vi "Network Parameters DAO.vi"(5 "Section":string="DataTransmission", 7 "refnum":T2, 8 "error in (no error)":errorcluster, 10 "Network Parameters In":T1={"Port Number"=0, "Notification Name"="DataAvailableForTransmission", "Wait For Notification Timeout"=1000}, 11 "Persistent DAO Actions":T3) -> (0 "error out":errorcluster, 3 "Network Parameters Out":T1={"Port Number"=0, "Notification Name"="DataAvailableForTransmission", "Wait For Notification Timeout"=1000}, 4 "refnum out":T2)   [LabVIEW 2013]
uses:
  Network Parameters.ctl
  Metadata/Persistant DAO Actions.ctl
  <vilib>/Utility/config.llb/Config Data RefNum.ctl
  <vilib>/Utility/config.llb/Read Key (U32).vi
  <vilib>/Utility/config.llb/Read Key (I32).vi
  <vilib>/Utility/config.llb/Read Key (String).vi
  <vilib>/Utility/config.llb/Write Key (U32).vi
  <vilib>/Utility/config.llb/Write Key (I32).vi
  <vilib>/Utility/config.llb/Write Key (String).vi
  <vilib>/Utility/config.llb/NI_LVConfig.lvlib
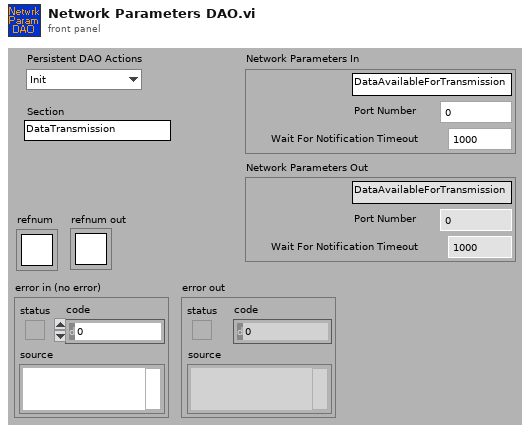
[diagram p1: front panel]
types:
  T1 = typedef "Network Parameters.ctl" = cluster{"Port Number":u16, "Notification Name":string, "Wait For Notification Timeout":i32}
  T2 = typedef "NI_LVConfig.lvlib/Config Data RefNum.ctl" = refnum<k1>
  T3 = typedef "Persistant DAO Actions.ctl" = enum16{"Init", "Get", "Set", "Load", "Save"}
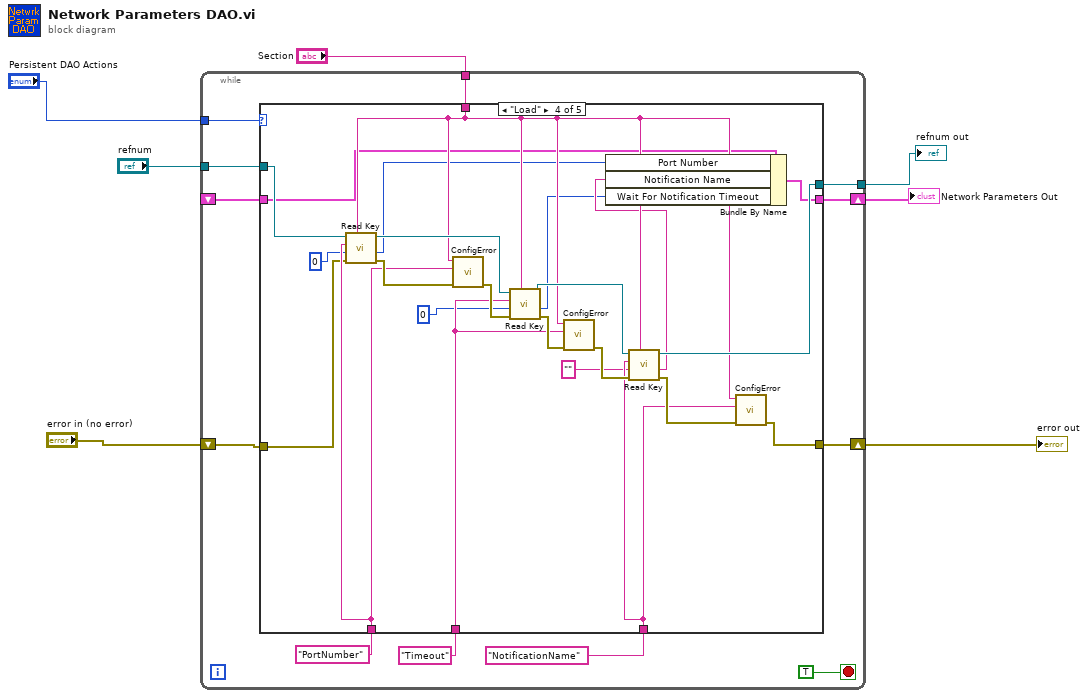
[diagram p0: block diagram]
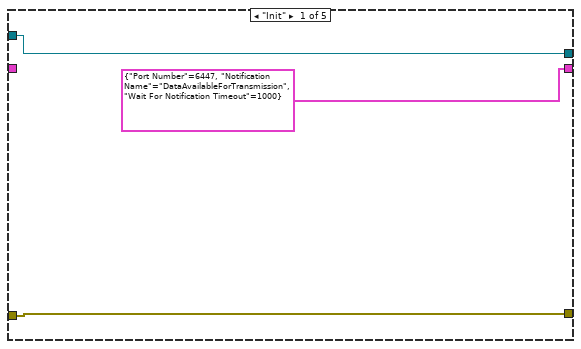
[diagram p2: hidden frame]
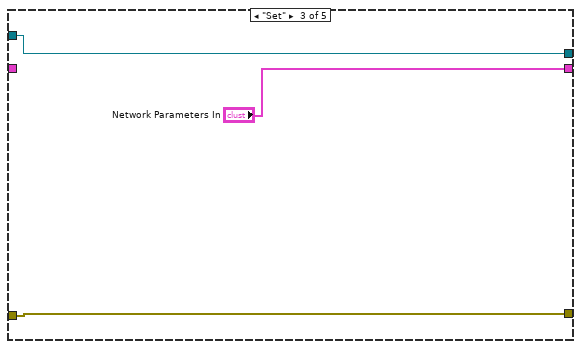
[diagram p4: hidden frame]
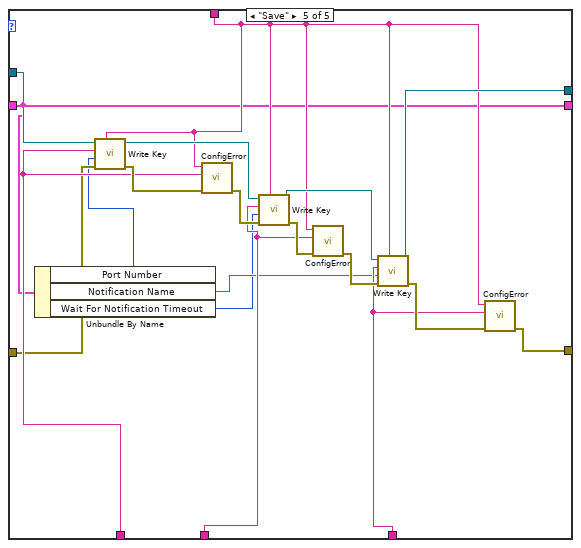
[diagram p5: hidden frame]
diagram:
  n1 = while {
    tunnel: "Persistent DAO Actions" -> [w18]
    shift-right: [w17] -> w6
    shift-left: _ -> [w16]
    tunnel: "refnum" -> [w14]
    shift-right: [w11] -> w3
    shift-left: "error in (no error)" -> [w12]
    tunnel: [w10] -> w2
    tunnel: "Section" -> [w8]
    stop <- TRUE stop-if-true
    n2 = case shown="\"Load\"" w18 {
      tunnel: [T1 {"Port Number"=6447, "Notification Name"="DataAvailableForTransmission", "Wait For Notification Timeout"=1000} ("Network Parameters In") w25 "Network Parameters In" w33 w54] -> w17
      tunnel: w16 -> [_ w25 _ w32 w54]
      tunnel: w8 -> [_ _ _ w38 w58]
      tunnel: "PortNumber" -> [_ _ _ w50 w69]
      tunnel: w14 -> [w22 w23 w27 w49 w68]
      tunnel: "Timeout" -> [_ _ _ w45 w64]
      tunnel: w12 -> [w21 w24 w28 w43 w63]
      tunnel: [w21 w24 w28 w35 w56] -> w11
      tunnel: [w22 w23 w27 w39 w59] -> w10
      tunnel: "NotificationName" -> [_ _ _ w37 w57]
      frame "Init" {
      }
      frame "Get" {
      }
      frame "Set" {
      }
      frame "Load" {
        n3 = call-poly <vilib>:"Read Key.vi"("section"=w38, "error in (no error)"=w43, "default value"=u16 0 ("Port Number In"), "key"=w50, "refnum"=w49) -> ("error out"=w51:errorcluster, "value"=w31:u32, "refnum out"=w46:T2)  [unwired: 4 out]
        n4 = call "ConfigError.vi"("error in (no error)"=w51, "Key"=w50, "Section"=w38) -> ("error out"=w47:errorcluster)  [unwired: 8 out]
        n5 = call-poly <vilib>:"Read Key.vi"("section"=w38, "error in (no error)"=w47, "default value"=0 ("Wait For Notification Timeout In"), "key"=w45, "refnum"=w46) -> ("error out"=w48:errorcluster, "value"=w29:i32, "refnum out"=w40:T2)  [unwired: 4 out]
        n6 = call "ConfigError.vi"("error in (no error)"=w48, "Key"=w45, "Section"=w38) -> ("error out"=w41:errorcluster)  [unwired: 8 out]
        n7 = call-poly <vilib>:"Read Key.vi"("section"=w38, "error in (no error)"=w41, "default value"="", "key"=w37, "refnum"=w40) -> ("error out"=w42:errorcluster, "value"=w30:string, "refnum out"=w39:T2)  [unwired: 1 in, 3 out]
        n8 = Bundle By Name(cluster=w32, "Port Number"=w31, "Notification Name"=w30, "Wait For Notification Timeout"=w29) -> (w33:T1)
        n9 = call "ConfigError.vi"("error in (no error)"=w42, "Key"=w37, "Section"=w38) -> ("error out"=w35:errorcluster)  [unwired: 8 out]
      }
      frame "Save" {
        n10 = Unbundle By Name(w54) -> ("Port Number"=w55:u16, "Notification Name"=w53:string, "Wait For Notification Timeout"=w52:i32)
        n11 = call-poly <vilib>:"Write Key.vi"("section"=w58, "error in (no error)"=w63, "value"=w55, "key"=w69, "refnum"=w68) -> ("error out"=w70:errorcluster, "refnum out"=w65:T2)  [unwired: 5 out]
        n12 = call "ConfigError.vi"("error in (no error)"=w70, "Key"=w69, "Section"=w58) -> ("error out"=w66:errorcluster)  [unwired: 8 out]
        n13 = call-poly <vilib>:"Write Key.vi"("section"=w58, "error in (no error)"=w66, "value"=w52, "key"=w64, "refnum"=w65) -> ("error out"=w67:errorcluster, "refnum out"=w60:T2)  [unwired: 5 out]
        n14 = call "ConfigError.vi"("error in (no error)"=w67, "Key"=w64, "Section"=w58) -> ("error out"=w61:errorcluster)  [unwired: 8 out]
        n15 = call-poly <vilib>:"Write Key.vi"("section"=w58, "error in (no error)"=w61, "value"=w53, "key"=w57, "refnum"=w60) -> ("error out"=w62:errorcluster, "refnum out"=w59:T2)  [unwired: 1 in, 4 out]
        n16 = call "ConfigError.vi"("error in (no error)"=w62, "Key"=w57, "Section"=w58) -> ("error out"=w56:errorcluster)  [unwired: 8 out]
      }
    }
  }
  "Network Parameters Out" <- w6
  "error out" <- w3
  "refnum out" <- w2
